vi "FT_Status to Error.vi"(8 "error in (no error)":errorcluster, 10 "FT_Status":u32) -> (0 "error out":errorcluster)   [LabVIEW 2019, in "D2XX-lv.lvlib"]
uses:
  D2XX-lv.lvlib
  D2XX_Functions_7.0/D2XX.lvlib
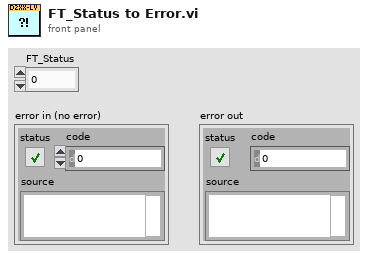
[diagram p1: front panel]
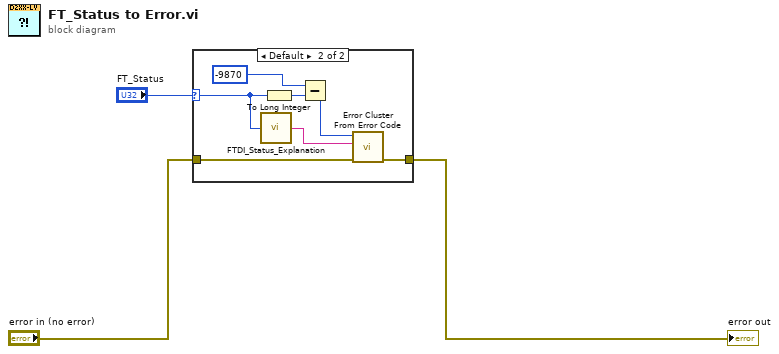
[diagram p0: block diagram]
diagram:
  n1 = case shown="Default" "FT_Status" {
    selector: "FT_Status" -> [_ w9]
    tunnel: "error in (no error)" -> [w4 w11]
    tunnel: [w4 w5] -> w2
    frame 0 {
    }
    frame Default {
      n2 = call "FTDI_Status_Explanation.vi"("FT_Status"=w9) -> ("Status String"=w10:string)
      n3 = To Long Integer(number=w9) -> (32bit integer=w6:i32)
      n4 = Subtract(x=-9870, y=w6) -> (x-y=w8:i32)
      n5 = call <vilib>:"Error Cluster From Error Code.vi"("error in (no error)"=w11, "error message (\"\")"=w10, "error code (0)"=w8) -> ("error out"=w5:errorcluster)  [unwired: 6 in]
    }
  }
  "error out" <- w2
